vi "4Columns.vi"   [LabVIEW 2015]
types:
  T1 = enum16{"open", "replace", "create", "open or create", "replace or create", "replace or create with confirmation"}
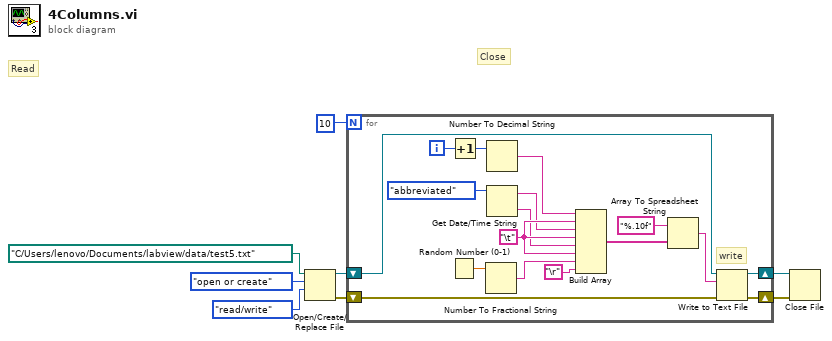
[diagram p0: block diagram]
diagram:
  # "Read"
  # "Close"
  n1 = Open/Create/Replace File(file path (use dialog)=path "C:/Users/lenovo/Documents/labview/data/test5.txt", operation (0:open)=T1."open or create", access (0:read/write)=enum16{"read/write", "read-only", "write-only"}."read/write") -> (refnum out=w4:refnum<file>, error out=w3:errorcluster)  [unwired: 3 in, 1 out]
  n2 = for {
    N: 10 -> [_]
    shift-right: [w22] -> w1
    shift-left: w4 -> [w25]
    shift-right: [w23] -> w2
    shift-left: w3 -> [w24]
    i -> [w16]
    w12 = "\t"
    # "write"
    n3 = Random Number (0-1)() -> (number: 0 to 1=w17:dbl)
    n4 = Increment(x=w16) -> (x+1=w15:i32)
    n5 = Number To Fractional String(number=w17) -> (F-format string=w13:string)  [unwired: 3 in]
    n6 = Number To Decimal String(number=w15) -> (decimal integer string=w21:string)  [unwired: 1 in]
    n7 = Get Date/Time String(date format (0)=enum16{"short", "long", "abbreviated"}."abbreviated") -> (date string=w9:string, time string=w10:string)  [unwired: 2 in]
    n8 = Build Array(w21, w12, w9, w12, w10, w12, w13, "\r") -> (w19:string[])
    n9 = Array To Spreadsheet String(array=w19, 3:"%.10f" ("format string")) -> (spreadsheet string=w18:string)  [unwired: 1 in]
    n10 = Write to Text File(file (use dialog)=w25, text=w18, error in=w24) -> (refnum out=w22:refnum<file>, error out=w23:errorcluster)  [unwired: 1 in, 1 out]
  }
  n11 = Close File(refnum=w1, error in=w2) -> ()  [unwired: 2 out]
